vi "sr830_setup_GPIB_9.vi"(2 "Lock In #2 Sensitivity":i32=15) -> ()   [LabVIEW 2016]
uses:
  Instrument_Setup.vi
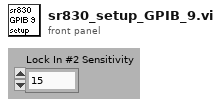
[diagram p1: front panel]
types:
  T1 = cluster{"sensitivity\n2nV/fA":i32, "dyn reserve\n(low noise:2)":i16, "ref. phase":ext, "automeasure":bool}
  T2 = cluster{"time constant\n(10 µs : 0) ":i32, "slope (6 dB/oct)":i32}
  T3 = cluster{" display":i32, " ratio":u16, "output":u16}
  T4 = cluster{"off. & exp.":u16, "offset":dbl, "expand":u16}
  T5 = cluster{"ref. source":bool, "osc.harm# ":u16, "osc. freq":ext, "osc. ampl.":ext, "ref. trigger":u16}
  T6 = cluster{"input":u16, "ground":bool, "couple":bool}
  T7 = cluster{"sync filter":bool, "line filter\n(off:0)":i32}
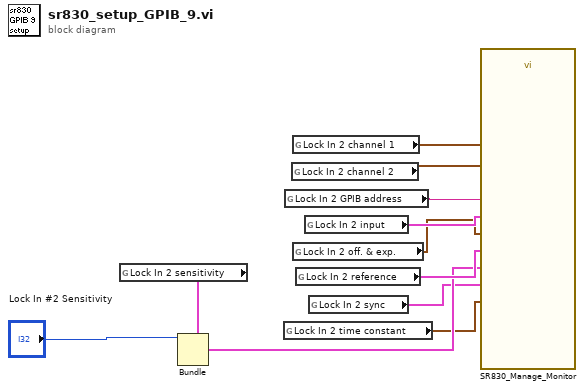
[diagram p0: block diagram]
diagram:
  n1 = global read "Instrument_Setup.vi" "Lock In 2 sensitivity"() -> (w4:T1)
  n2 = Bundle(cluster=w4, "sensitivity\n2nV/fA"="Lock In #2 Sensitivity") -> (w3:T1)  [unwired: 3 in]
  n3 = global read "Instrument_Setup.vi" "Lock In 2 time constant"() -> (w1:T2)
  n4 = global read "Instrument_Setup.vi" "Lock In 2 GPIB address"() -> (w8:string)
  n5 = global read "Instrument_Setup.vi" "Lock In 2 channel 2"() -> (w9:T3)
  n6 = global read "Instrument_Setup.vi" "Lock In 2 channel 1"() -> (w10:T3)
  n7 = global read "Instrument_Setup.vi" "Lock In 2 off. & exp."() -> (w6:T4)
  n8 = global read "Instrument_Setup.vi" "Lock In 2 reference"() -> (w5:T5)
  n9 = global read "Instrument_Setup.vi" "Lock In 2 input"() -> (w7:T6)
  n10 = global read "Instrument_Setup.vi" "Lock In 2 sync"() -> (w2:T7)
  n11 = call "SR830_Manage_Monitor.vi"("GPIB address"=w8, "input"=w7, "channel 1"=w10, "sensitivity"=w3, "sync"=w2, "reference"=w5, "time constant"=w1, "off. & exp."=w6, "channel 2"=w9) -> ()  [unwired: 4 in, 3 out]
